vi "Has Destroyed.vi"(7 "Sender":refnum<class "Sender.lvclass">, 9 "Error":errorcluster, 10 "Actor":refnum<class "Actor.lvclass">) -> (2 "Msg":refnum<class "Msg.lvclass">)   [LabVIEW 2020, in "jettl.lvlib" / "Has Destroyed Msg.lvlib"]
uses:
  Has Destroyed Msg.lvlib
  Msg/Msg.lvclass
  Actor/Actor/Actor.lvclass
  Sender/Sender/Sender.lvclass
  Has Destroyed Msg/Has Destroyed Msg.lvclass
  C:/git/jettl/src/jettl/jettl/Msg/Msg.lvclass
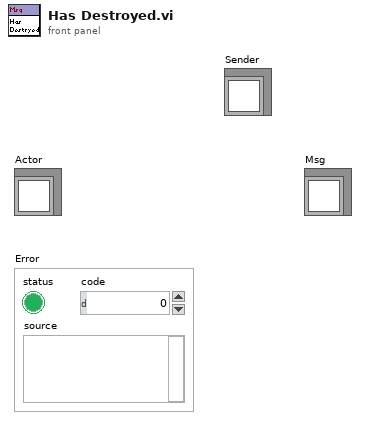
[diagram p1: front panel]
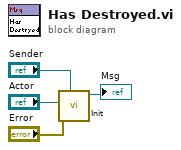
[diagram p0: block diagram]
diagram:
  n1 = call "Init.vi"("Sender"="Sender", "Error"="Error", "Actor"="Actor") -> ("Has Destroyed Msg out"=→"Msg":refnum<class "Has Destroyed Msg.lvclass">)  [unwired: 8 in]
